vi "Eratosthenes sieve.vi"() -> ()   [LabVIEW 2021]
panel:
  out "Array 2":dbl[](array[numeric])
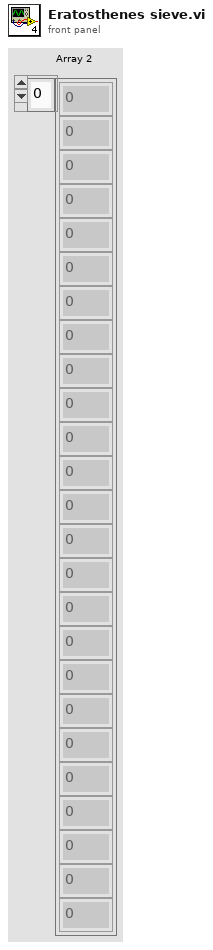
[diagram p1: front panel]
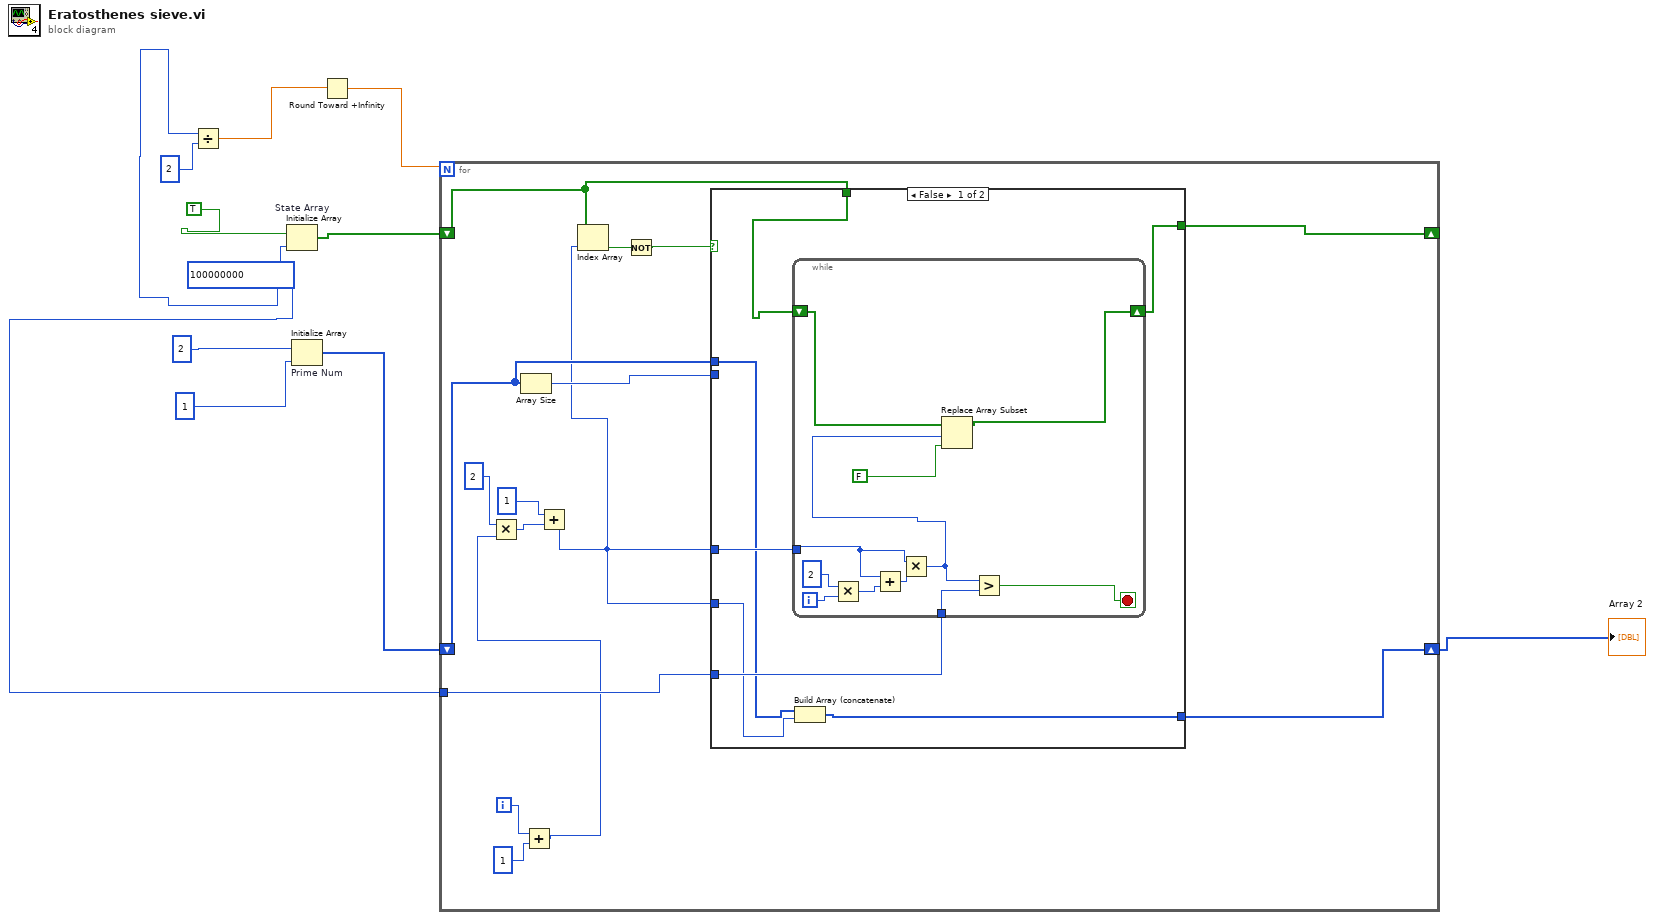
[diagram p0: block diagram]
diagram:
  w5 = 100000000
  n1 = Divide(x=w5, y=2) -> (x/y=w3:dbl)
  n2 = Initialize Array "State Array"(TRUE, w5) -> (w8:bool[])
  n3 = Initialize Array "Prime Num"(2, 1) -> (w7:i32[])
  n4 = Round Toward +Infinity(x=w3) -> (ceil(x): smallest int >= x=w2:dbl)
  n5 = for {
    N: w2 -> [_]
    shift-right: [w16] -> _
    shift-left: w8 -> [w17]
    shift-right: [w20] -> w4
    shift-left: w7 -> [w22]
    tunnel: w5 -> [w18]
    i -> [w15]
    n6 = Array Size(array=w22) -> (size(s)=w21:i32)
    n7 = Add(x=w15, y=1) -> (x+y=w13:i32)
    n8 = Multiply(x=2, y=w13) -> (x*y=w24:i32)
    n9 = Add(x=1, y=w24) -> (x+y=w19:i32)
    n10 = Index Array(array=w17, index=w19) -> (element=w11:bool)
    n11 = Not(x=w11) -> (.not. x?=w12:bool)
    n12 = case shown="False" w12 {
      tunnel: w22 -> [w27 w44]
      tunnel: w19 -> [w26 _]
      tunnel: w21 -> [_ _]
      tunnel: [w28 w44] -> w20
      tunnel: w19 -> [w32 _]
      tunnel: w18 -> [w31 _]
      tunnel: w17 -> [w30 w45]
      tunnel: [w29 w45] -> w16
      frame False {
        n13 = while {
          tunnel: w32 -> [w39]
          tunnel: w31 -> [w37]
          shift-right: [w34] -> w29
          shift-left: w30 -> [w36]
          i -> [w43]
          stop <- w38 stop-if-true
          n14 = Multiply(x=2, y=w43) -> (x*y=w41:i32)
          n15 = Add(x=w39, y=w41) -> (x+y=w40:i32)
          n16 = Multiply(x=w39, y=w40) -> (x*y=w35:i32)
          n17 = Replace Array Subset(array=w36, new element=FALSE, index=w35) -> (w34:bool[])
          n18 = Greater?(x=w35, y=w37) -> (0:w38:bool)
        }
        n19 = Build Array (concatenate)(w27, w26) -> (w28:i32[])
      }
      frame True {
      }
    }
  }
  "Array 2" <- w4
